vi "arduino-Labview.vi"() -> ()   [LabVIEW 2020]
uses:
  <vilib>/LabVIEW Interface for Arduino/LabVIEW Interface for Arduino.lvlib
panel:
  in  "Tab Control":enum32{"Page 1", "Page 2"}(tab)
  in  "stop":bool
  in  "VISA resource":refnum<visa-resource-name>
  in  "Digital I/O Pin (0)":u8
  in  "Boolean":bool
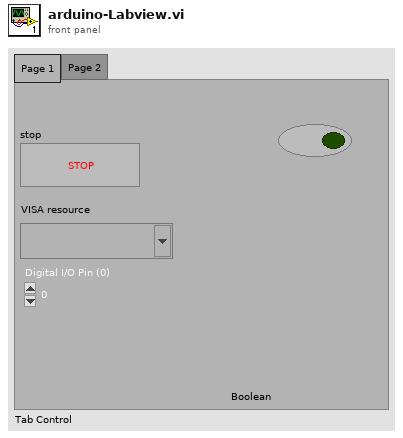
[diagram p1: front panel]
types:
  T1 = typedef "LabVIEW Interface for Arduino.lvlib/Arduino Resource.ctl" = cluster{"VISA resource":refnum<visa-resource-name>, "Board Type":T2, "Connection Type":enum8{"USB / Serial"}, "Bytes Per Packet (15)":u8}
  T2 = typedef "LabVIEW Interface for Arduino.lvlib/Board Type.ctl" = enum16{"Uno", "Dimuelanove w/Atmega 328", "Mega 2560"}
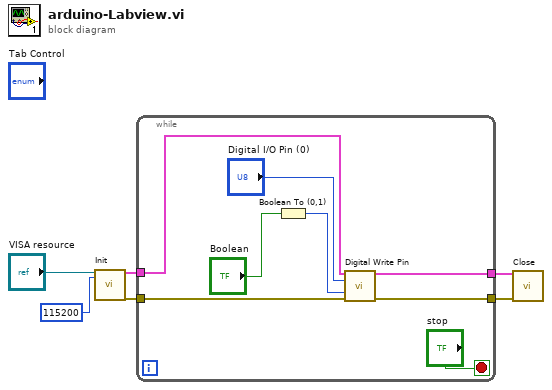
[diagram p0: block diagram]
diagram:
  n1 = call <vilib>:"Init.vi"("VISA resource"="VISA resource", "Baud Rate (115200)"=u32 115200) -> ("Arduino Resource"=w6:T1, "error out"=w3:errorcluster)  [unwired: 16 in]
  n2 = while {
    tunnel: w6 -> [w14]
    tunnel: [w13] -> w5
    tunnel: [w12] -> w4
    tunnel: w3 -> [w10]
    stop <- "stop" stop-if-true
    n3 = Boolean To (0,1)(Boolean="Boolean") -> (0, 1=w8:i16)
    n4 = call <vilib>:"Digital Write Pin.vi"("Arduino Resource"=w14, "Digital I/O Pin (0)"="Digital I/O Pin (0)", "Value (0)"=w8, "error in"=w10) -> ("Arduino Resource"=w13:T1, "error out"=w12:errorcluster)  [unwired: 10 in]
  }
  n5 = call <vilib>:"Close.vi"("Arduino Resource"=w5, "error in"=w4) -> ()  [unwired: 13 in, 1 out]
